vi "MultiFreqVelocityMove.vi"() -> ()   [LabVIEW 2022 SP3]
uses:
  <vilib>/Motion/FlexMotion/FunctionsVIs/Trajectory.llb/Load Acceleration/Deceleration.flx
  <vilib>/measure/NI_MAPro.lvlib
  <vilib>/Motion/FlexMotion/FunctionsVIs/StartStopMotion.llb/Start Motion (8 axes).flx
  <vilib>/Motion/FlexMotion/FunctionsVIs/StartStopMotion.llb/Stop Motion (8 axes).flx
  <vilib>/Utility/file.llb/Write Delimited Spreadsheet (DBL).vi
  <vilib>/Motion/FlexMotion/CustomControls/CustomControls.llb/Mask (8 axes).flx
  <vilib>/Motion/FlexMotion/FunctionsVIs/MotionIO.llb/Set Breakpoint Output MOMO (8 axes).flx
  <vilib>/Motion/FlexMotion/FunctionsVIs/Trajectory.llb/Wait for Move Complete (8 axes).flx
  <vilib>/Motion/FlexMotion/CustomControls/CustomControls.llb/AxisOrVectorSpace To Control.flx
panel:
  out "Final Position":i32
  out "Position":i32
  out "error out":errorcluster
  in  "Position Trigger Out?":bool=TRUE
  in  "Trigger every X Revolutions?":dbl=1.0
  in  "Filename":path=path "F:/test.txt"
  out "Filename Out":path=path "F:/test.txt"
  in  "Save Motor Velocities?":bool caption="Enable"
  in  "System Initilized?":bool
  in  "Stop":bool
  out "XY Graph":cluster{dbl[], dbl[]}[](graph)
  in  "Number of Components":i8=1 min=1 step=1
  in  "Seconds of Run Time":dbl=30.0
  in  "Counts Per (mm or rotation)":dbl=4000.0
  in  "Axis or Vector Space":T1=2 caption="Axis" items=["Axis 1"=1, "Axis 2"=2, "Axis 3"=3, "Axis 4"=4, "Axis 5"=5, "Axis 6"=6, "Axis 7"=7, "Axis 8"=8, "Vector Space 1"=17, "Vector Space 2"=18, "Vector Space 3"=19, "Vector Space 4"=20]
  in  "Component Phases":dbl[](array[numeric])=[0.0, 0.0, 0.0, 0.0] format="%.2p"
  in  "Component Speeds ((mm or rotations)/s)":dbl[](array[numeric])=[1.0, 0.25, 0.25, 1.0] format="%.2p"
  in  "Component Freqs (Hz)":dbl[](array[numeric])=[0.0, 5.0, 10.0, 400.0]
  in  "Run":bool
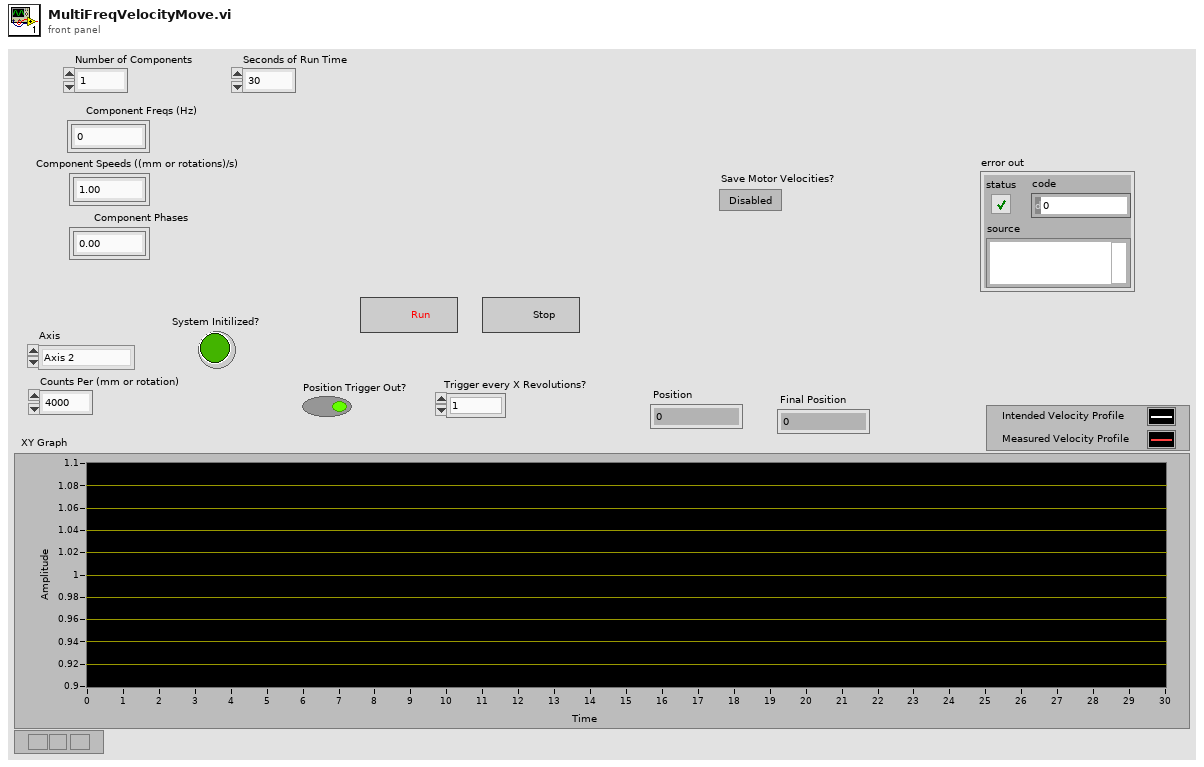
[diagram p1: front panel]
types:
  T1 = typedef "AxisOrVectorSpace To Control.flx" = u16
  T2 = typedef "Bd Id Out" = u8
  T3 = typedef "Mask (8 axes).flx" = cluster{"1":bool, "2":bool, "3":bool, "4":bool, "5":bool, "6":bool, "7":bool, "8":bool}
  T4 = enum16{"Absolute Position", "Relative Position", "Velocity", "Relative to Cap Pos", "Modulus Position", "Absolute Contouring", "Relative Contouring"}
  T5 = typedef "BoardID.ctl" = i32
  T6 = typedef "Resource Out (Enum).flx" = u16
  T7 = enum16{"No Change", "Reset on Breakpoint", "Set on Breakpoint", "Toggle on Breakpoint", "Create Pulse on Breakpoint"}
  T8 = enum16{"Absolute Breakpoint", "Relative Breakpoint", "Modulo Breakpoint", "Periodic Breakpoint"}
  T9 = enum16{"open", "replace", "create", "open or create", "replace or create", "replace or create with confirmation"}
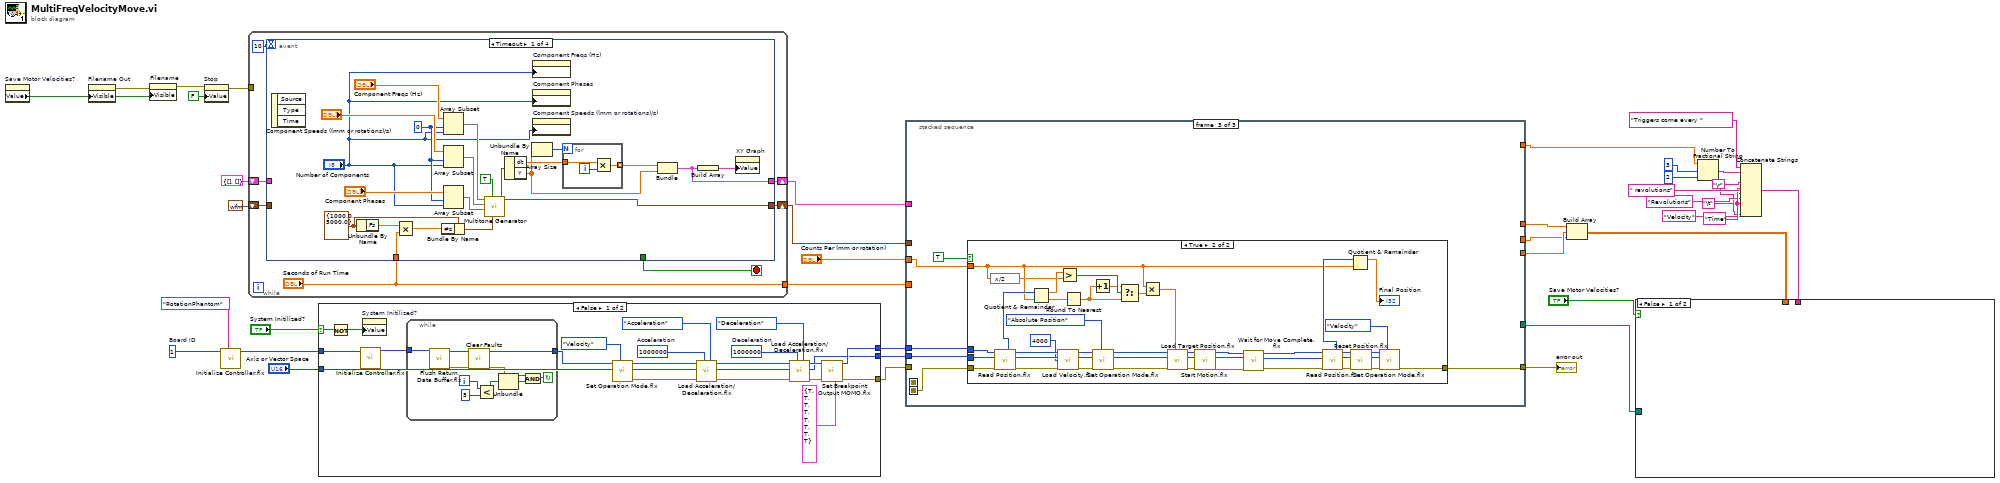
[diagram p0: block diagram]
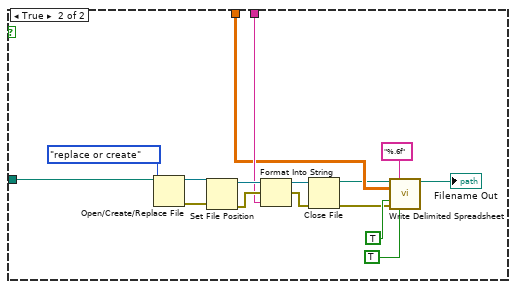
[diagram p2: hidden frame]
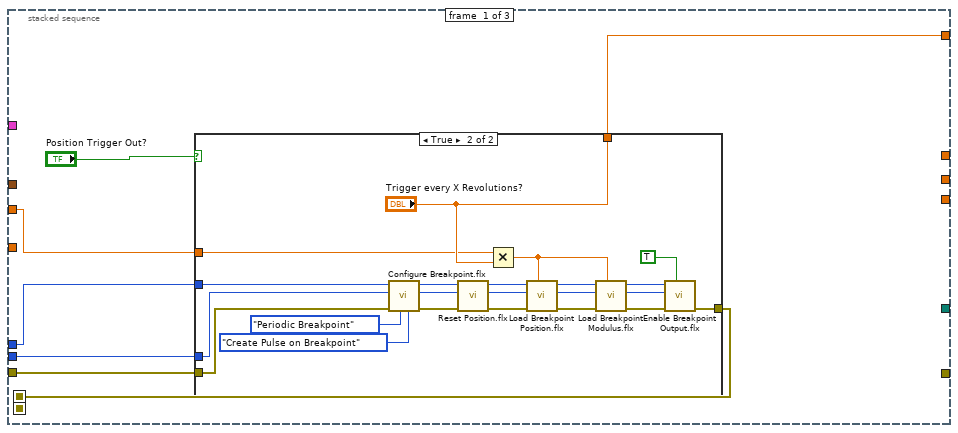
[diagram p3: hidden frame]
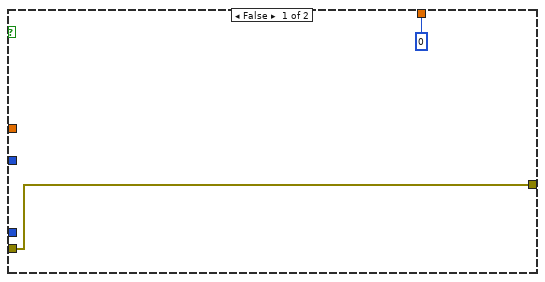
[diagram p4: hidden frame]
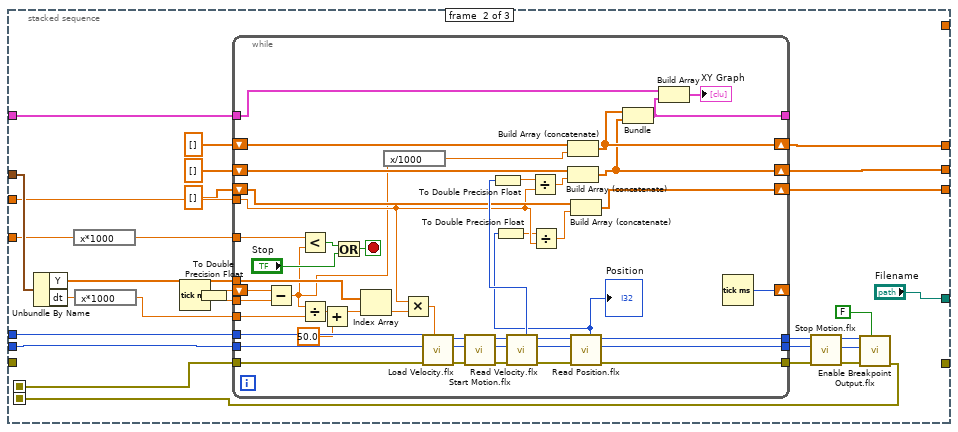
[diagram p5: hidden frame]
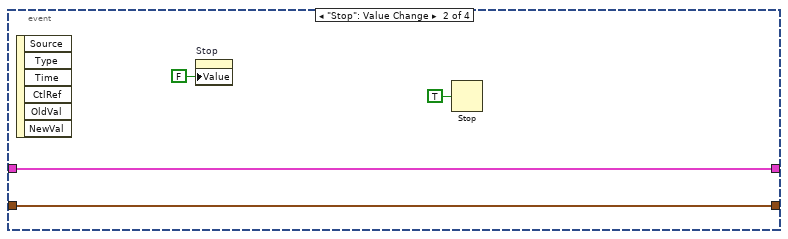
[diagram p8: hidden frame]
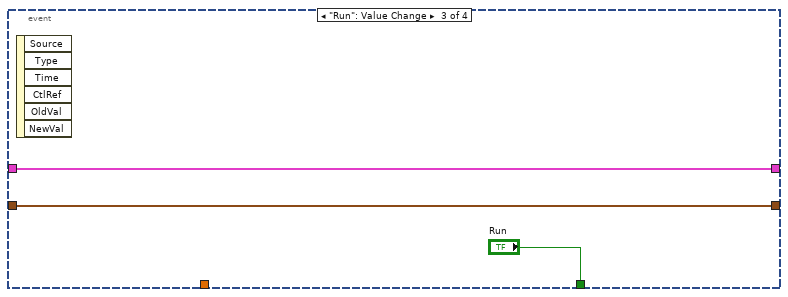
[diagram p9: hidden frame]
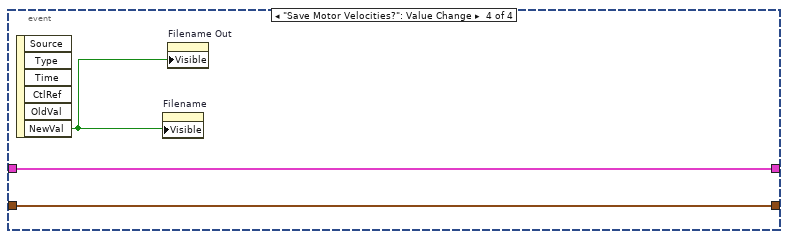
[diagram p10: hidden frame]
diagram:
  w8 = "\t"
  w9 = "\r"
  w2 = u8 1  # Board ID
  n1 = property on="Save Motor Velocities?" class="Bool (strict)"() -> ("Value"=w26:bool)  [unwired: 2 in, 2 out]
  n2 = property on="Filename Out" class="Path"("Visible"=w26) -> (error out=w25:errorcluster)  [unwired: 2 in, 1 out]
  n3 = property on="Filename" class="Path"(error in=w25, "Visible"=w26) -> (error out=w24:errorcluster)  [unwired: 1 in, 1 out]
  n4 = property on="Stop" class="Bool (strict)"(error in=w24, "Value"=FALSE ("Stop")) -> (error out=w14:errorcluster)  [unwired: 1 in, 1 out]
  n5 = call <vilib>:"Initialize Controller.flx"("Settings Name"="RotationPhantom", "Board ID"=w2) -> ("Bd ID Out"=w1:T2)  [unwired: 6 in, 1 out]
  n6 = while {
    tunnel: ["Seconds of Run Time"] -> w38
    shift-right: [w44] -> w36
    shift-left: cluster{dbl[], "Y":dbl[]} {[], "Y"=[]} -> [w43]
    shift-right: [w45] -> w37
    shift-left: waveform(dbl) {"t0"=timestamp(0 s since 1904-01-01), "dt"=1.0, "Y"=[]} ("signal out") -> [w42]
    tunnel: w14 -> [_]
    stop <- w40 stop-if-true
    n7 = event shown="[0] Timeout" {
      selector: _ -> [_ _ _ _]
      dyn-events: _ -> [_ _ _ _]
      timeout: 10 -> [_ _ _ _]
      tunnel: "Seconds of Run Time" -> [w46 _ _ _]
      tunnel: [w55 w73 w76 w79] -> w45
      tunnel: [w49 w72 w75 w78] -> w44
      tunnel: w43 -> [_ w72 w75 w78]
      tunnel: w42 -> [_ w73 w76 w79]
      tunnel: [_ _ "Run" _] -> w40
      event Timeout {
        w56 = 0 ("index")
        w63 = cluster{"Fs":dbl, "#s":dbl} {"Fs"=1000.0, "#s"=5000.0} ("sampling info")
        n8 = event-data() -> ()  [unwired: 1 in, 3 out]
        n9 = Unbundle By Name(w63) -> ("Fs"=w60:dbl)
        n10 = Multiply(x=w60, y=w46) -> (x*y=w62:dbl)
        n11 = Bundle By Name(cluster=w63, "#s"=w62) -> (w61:cluster{"Fs":dbl, "#s":dbl})
        n12 = Array Subset(array="Component Freqs (Hz)", index=w56, length="Number of Components") -> (w59:dbl[])
        n13 = Array Subset(array="Component Speeds ((mm or rotations)/s)", index=w56, length="Number of Components") -> (w58:dbl[])
        n14 = Array Subset(array="Component Phases", index=w56, length="Number of Components") -> (w57:dbl[])
        n15 = call <vilib>:"Multitone Generator.vi"("sampling info"=w61, "reset signal"=TRUE, "tone phases"=w57, "tone amplitudes"=w58, "tone frequencies"=w59) -> ("signal out"=w55:waveform(dbl))  [unwired: 3 in, 3 out]
        n16 = Unbundle By Name(w55) -> ("dt"=w54:dbl, "Y"=w50:dbl[])
        n17 = Array Size(array=w50) -> (size(s)=w51:i32)
        n18 = property on="Component Freqs (Hz)" class="Arr (strict)"("Number of Columns"="Number of Components") -> ()  [unwired: 2 in, 2 out]
        n19 = property on="Component Phases" class="Arr (strict)"("Number of Columns"="Number of Components") -> ()  [unwired: 2 in, 2 out]
        n20 = property on="Component Speeds ((mm or rotations)/s)" class="Arr (strict)"("Number of Columns"="Number of Components") -> ()  [unwired: 2 in, 2 out]
        n21 = for {
          N: w51 -> [_]
          tunnel: w54 -> [w68]
          tunnel: [w67] -> w53 mode=indexing
          i -> [w69]
          n22 = Multiply(x=w68, y=w69) -> (x*y=w67:dbl)
        }
        n23 = Bundle(w53, "Y"=w50) -> (w49:cluster{dbl[], "Y":dbl[]})  [unwired: 1 in]
        n24 = Build Array(w49) -> (w52:cluster{dbl[], "Y":dbl[]}[])
        n25 = property on="XY Graph" class="XYGraph (strict)"("Value"=w52) -> ()  [unwired: 2 in, 2 out]
      }
      event "Stop": Value Change {
        n26 = event-data() -> ()  [unwired: 1 in, 6 out]
        n27 = property on="Stop" class="Bool (strict)"("Value"=FALSE ("Stop")) -> ()  [unwired: 2 in, 2 out]
        n28 = Stop(stop? (T)=TRUE) -> ()
      }
      event "Run": Value Change {
        n29 = event-data() -> ()  [unwired: 1 in, 6 out]
      }
      event "Save Motor Velocities?": Value Change {
        n30 = event-data() -> ("NewVal"=w77:bool)  [unwired: 1 in, 5 out]
        n31 = property on="Filename" class="Path"("Visible"=w77) -> ()  [unwired: 2 in, 2 out]
        n32 = property on="Filename Out" class="Path"("Visible"=w77) -> ()  [unwired: 2 in, 2 out]
      }
    }
  }
  n33 = case shown="False" "System Initilized?" {
    selector: "System Initilized?" -> [w102 _]
    tunnel: [w83 w114] -> w31
    tunnel: "Axis or Vector Space" -> [w86 w114]
    tunnel: w1 -> [w100 w113]
    tunnel: [w84 w113] -> w32
    tunnel: [w80 _] -> w30
    frame False {
      w94 = u32 1000000  # Deceleration
      w93 = u32 1000000  # Acceleration
      n34 = Not(x=w102) -> (.not. x?=w101:bool)
      n35 = call <vilib>:"Initialize Controller.flx"("Board ID"=w100) -> ("Bd ID Out"=w99:T2)  [unwired: 7 in, 1 out]
      n36 = property on="System Initilized?" class="Bool (strict)"("Value"=w101) -> ()  [unwired: 2 in, 2 out]
      n37 = while {
        tunnel: w99 -> [w112]
        tunnel: [w110] -> w87
        i -> [w105]
        stop <- w106 continue-if-true
        n38 = call <vilib>:"Flush Return Data Buffer.flx"("Board ID"=w112) -> ("error out"=w108:errorcluster, "Bd ID Out"=w111:T2)  [unwired: 6 in]
        n39 = call <vilib>:"Clear Faults.vi"("error in (no error)"=w108, "board in"=w111) -> ("error out"=w109:errorcluster, "board out"=w110:T5)  [unwired: 8 in]
        n40 = Less?(x=w105, y=5) -> (x < y?=w104:bool)
        n41 = Unbundle(w109) -> ("status"=w107:bool)  [unwired: 2 out]
        n42 = And(x=w107, y=w104) -> (x .and. y?=w106:bool)
      }
      n43 = call <vilib>:"Set Operation Mode.flx"("Position Mode (Absolute)"=T4."Velocity", "Axis or Vector Space"=w86, "Board ID"=w87) -> ("error out"=w98:errorcluster, "Resource Output"=w96:T6, "Bd ID Out"=w97:T2)  [unwired: 3 in]
      n44 = call "Load Acceleration/Deceleration.flx"("Acceleration Type (Both)"=enum16{"Both", "Acceleration", "Deceleration"}."Acceleration", "Acceleration (100000)"=w93, "error in (no error)"=w98, "Axis or Vector Space"=w96, "Board ID"=w97) -> ("error out"=w90:errorcluster, "Resource Output"=w88:T6, "Bd ID Out"=w89:T2)  [unwired: 2 in]
      n45 = call "Load Acceleration/Deceleration.flx"("Acceleration Type (Both)"=enum16{"Both", "Acceleration", "Deceleration"}."Deceleration", "Acceleration (100000)"=w94, "error in (no error)"=w90, "Axis or Vector Space"=w88, "Board ID"=w89) -> ("error out"=w81:errorcluster, "Resource Output"=w83:T6, "Bd ID Out"=w85:T2)  [unwired: 2 in]
      n46 = call-poly <vilib>:"Set Breakpoint Output MOMO.flx"("Must Off (False)"=T3 {"1"=TRUE, "2"=TRUE, "3"=TRUE, "4"=TRUE, "5"=TRUE, "6"=TRUE, "7"=TRUE, "8"=TRUE}, "error in (no error)"=w81, "Board ID"=w85) -> ("error out"=w80:errorcluster, "Bd ID Out"=w84:T2)  [unwired: 3 in, 2 out]
    }
    frame True {
    }
  }
  n47 = stacked-sequence {
    seq-local: [w115 _ _] -> [_ w150 _]
    seq-local: [_ w146 _] -> [_ _ w223]
    tunnel: w37 -> [_ w173 _]
    tunnel: w32 -> [w121 w148 w226]
    tunnel: w31 -> [w120 w147 w225]
    tunnel: w30 -> [w119 _ _]
    tunnel: w38 -> [_ w169 _]
    tunnel: w36 -> [_ w165 _]
    tunnel: "Counts Per (mm or rotation)" -> [w116 w163 w224]
    tunnel: [_ w160 _] -> w23
    tunnel: [_ w159 _] -> w21
    tunnel: [_ w152 _] -> w22
    tunnel: [w117 _ _] -> w19
    tunnel: [_ "Filename" _] -> w6
    tunnel: [_ _ w222] -> w4
    frame #0 {
      n48 = case shown="True" "Position Trigger Out?" {
        tunnel: w121 -> [_ w125]
        tunnel: w120 -> [_ w124]
        tunnel: w119 -> [w122 w140]
        tunnel: [0 ("Breakpoint Modolus") "Trigger every X Revolutions?"] -> w117
        tunnel: w116 -> [_ w127]
        tunnel: [w122 w126] -> w115
        frame False {
        }
        frame True {
          n49 = call <vilib>:"Configure Breakpoint.flx"("Action (No Change)"=T7."Create Pulse on Breakpoint", "Mode (Absolute)"=T8."Periodic Breakpoint", "error in (no error)"=w140, "Axis or Encoder"=w124, "Board ID"=w125) -> ("error out"=w134:errorcluster, "Resource Output"=w135:T6, "Bd ID Out"=w138:T2)  [unwired: 4 in]
          n50 = call <vilib>:"Reset Position.flx"("error in (no error)"=w134, "Axis"=w135, "Board ID"=w138) -> ("error out"=w133:errorcluster, "Resource Output"=w136:T6, "Bd ID Out"=w137:T2)  [unwired: 4 in]
          n51 = Multiply(x=w127, y="Trigger every X Revolutions?") -> (x*y=w128:dbl)
          n52 = call <vilib>:"Load Breakpoint Position.flx"("Breakpoint Position (0)"=w128, "error in (no error)"=w133, "Axis or Encoder"=w136, "Board ID"=w137) -> ("error out"=w139:errorcluster, "Resource Output"=w143:T6, "Bd ID Out"=w144:T2)  [unwired: 3 in]
          n53 = call <vilib>:"Load Breakpoint Modulus.flx"("Breakpoint Modulus (0)"=w128, "error in (no error)"=w139, "Axis or Encoder"=w143, "Board ID"=w144) -> ("error out"=w145:errorcluster, "Resource Output"=w141:T6, "Bd ID Out"=w142:T2)  [unwired: 3 in]
          n54 = call <vilib>:"Enable Breakpoint Output.flx"("Enable Breakpoint"=TRUE, "error in (no error)"=w145, "Axis or Encoder"=w141, "Board ID"=w142) -> ("error out"=w126:errorcluster)  [unwired: 3 in, 2 out]
        }
      }
    }
    frame #1 {
      n55 = Unbundle By Name(w173) -> ("Y"=w166:dbl[], "dt"=w161:dbl)
      n56 = expression code="x*1000"(w169) -> (w168:dbl)
      n57 = expression code="x*1000"(w161) -> (w167:dbl)
      n58 = Tick Count (ms)() -> (millisecond timer value=w170:u32)
      n59 = To Double Precision Float(number=w170) -> (double precision float=w149:dbl)
      n60 = while {
        tunnel: [w185] -> w171
        tunnel: [w184] -> w172
        tunnel: w150 -> [w216]
        tunnel: w147 -> [w220]
        tunnel: w148 -> [w190]
        tunnel: w166 -> [w215]
        tunnel: w167 -> [w211]
        shift-right: [w214] -> _
        shift-left: w149 -> [w213]
        tunnel: w149 -> [w212]
        tunnel: w168 -> [w208]
        tunnel: w165 -> [w203]
        shift-right: [w198] -> w160
        shift-left: dbl[] [] -> [w202]
        shift-right: [w197] -> w159
        shift-left: dbl[] [] -> [w201]
        tunnel: w163 -> [w180]
        tunnel: [w191] -> _
        tunnel: [w186] -> w154
        shift-right: [w183] -> w152
        shift-left: dbl[] [] -> [w182]
        stop <- w194 stop-if-true
        n61 = Subtract(x=w213, y=w212) -> (x-y=w176:dbl)
        n62 = Less?(x=w208, y=w176) -> (x < y?=w209:bool)
        n63 = Divide(x=w176, y=w211) -> (x/y=w195:dbl)
        n64 = Add(x=w195, y=50.0) -> (x+y=w178:dbl)
        n65 = Or(x=w209, y="Stop") -> (x .or. y?=w194:bool)
        n66 = Index Array(array=w215, index=w178) -> (element=w210:dbl)
        n67 = expression code="x/1000"(w176) -> (w192:dbl)
        n68 = Multiply(x=w180, y=w210) -> (x*y=w204:dbl)
        n69 = call <vilib>:"Load Velocity.flx"("Velocity (10000)"=w204, "error in (no error)"=w216, "Axis or Vector Space"=w220, "Board ID"=w190) -> ("error out"=w217:errorcluster, "Resource Output"=w219:T6, "Bd ID Out"=w218:T2)  [unwired: 3 in]
        n70 = call-poly <vilib>:"Start Motion.flx"("error in (no error)"=w217, "Axis or Vector Space"=w219, "Board ID"=w218) -> ("error out"=w205:errorcluster, "Resource Output"=w206:T6, "Bd ID Out"=w207:T2)  [unwired: 3 in]
        n71 = call <vilib>:"Read Velocity.flx"("error in (no error)"=w205, "Axis or Vector Space"=w206, "Board ID"=w207) -> ("error out"=w187:errorcluster, "Resource Output"=w188:T6, "Bd ID Out"=w189:T2, "Filtered Velocity"=w196:i32)  [unwired: 3 in]
        n72 = To Double Precision Float(number=w196) -> (double precision float=w175:dbl)
        n73 = Divide(x=w175, y=w180) -> (x/y=w200:dbl)
        n74 = Build Array (concatenate)(w202, w192) -> (w198:dbl[])
        n75 = Build Array (concatenate)(w201, w200) -> (w197:dbl[])
        n76 = call <vilib>:"Read Position.flx"("error in (no error)"=w187, "Axis"=w188, "Board ID"=w189) -> ("error out"=w186:errorcluster, "Resource Output"=w185:T6, "Bd ID Out"=w184:T2, "Position"=w179:i32)  [unwired: 3 in]
        "Position" <- w179
        n77 = To Double Precision Float(number=w179) -> (double precision float=w174:dbl)
        n78 = Divide(x=w174, y=w180) -> (x/y=w181:dbl)
        n79 = Build Array (concatenate)(w182, w181) -> (w183:dbl[])
        n80 = Bundle(w198, w197) -> (w191:cluster{dbl[], dbl[]})  [unwired: 1 in]
        n81 = Build Array(w203, w191) -> (→"XY Graph":cluster{dbl[], "Y":dbl[]}[])
        n82 = Tick Count (ms)() -> (millisecond timer value=w214:u32)
      }
      n83 = call-poly <vilib>:"Stop Motion.flx"("error in (no error)"=w154, "Axis or Vector Space"=w171, "Board ID"=w172) -> ("error out"=w156:errorcluster, "Resource Output"=w157:T6, "Bd ID Out"=w158:T2)  [unwired: 4 in]
      n84 = call <vilib>:"Enable Breakpoint Output.flx"("Enable Breakpoint"=FALSE, "error in (no error)"=w156, "Axis or Encoder"=w157, "Board ID"=w158) -> ("error out"=w146:errorcluster)  [unwired: 3 in, 2 out]
    }
    frame #2 {
      n85 = case shown="True" TRUE {
        tunnel: w226 -> [_ w269]
        tunnel: w225 -> [_ w268]
        tunnel: w224 -> [_ w238]
        tunnel: w223 -> [w227 w242]
        tunnel: [w227 w241] -> w222
        frame False {
        }
        frame True {
          n86 = expression code="x/2"(w238) -> (w237:dbl)
          n87 = call <vilib>:"Read Position.flx"("error in (no error)"=w242, "Axis"=w268, "Board ID"=w269) -> ("error out"=w255:errorcluster, "Resource Output"=w251:T6, "Bd ID Out"=w256:T2, "Position"=w267:i32)  [unwired: 3 in]
          n88 = Quotient & Remainder(x=w267, y=w238) -> (x-y*floor(x/y)=w239:dbl, floor(x/y)=w240:dbl)
          n89 = call <vilib>:"Load Velocity.flx"("Velocity (10000)"=4000, "error in (no error)"=w255, "Axis or Vector Space"=w251, "Board ID"=w256) -> ("error out"=w253:errorcluster, "Resource Output"=w252:T6, "Bd ID Out"=w254:T2)  [unwired: 3 in]
          n90 = Greater?(x=w239, y=w237) -> (0:w235:bool)
          n91 = Round To Nearest(number=w240) -> (nearest integer value=w234:dbl)
          n92 = Increment(x=w234) -> (x+1=w233:dbl)
          n93 = call <vilib>:"Set Operation Mode.flx"("Position Mode (Absolute)"=T4."Absolute Position", "error in (no error)"=w253, "Axis or Vector Space"=w252, "Board ID"=w254) -> ("error out"=w259:errorcluster, "Resource Output"=w263:T6, "Bd ID Out"=w266:T2)  [unwired: 2 in]
          n94 = Select(t=w233, s=w235, f=w234) -> (s? t:f=w236:dbl)
          n95 = Multiply(x=w238, y=w236) -> (x*y=w248:dbl)
          n96 = call <vilib>:"Load Target Position.flx"("Target Position (0)"=w248, "error in (no error)"=w259, "Axis"=w263, "Board ID"=w266) -> ("error out"=w258:errorcluster, "Resource Output"=w264:T6, "Bd ID Out"=w265:T2)  [unwired: 3 in]
          n97 = call-poly <vilib>:"Start Motion.flx"("error in (no error)"=w258, "Axis or Vector Space"=w264, "Board ID"=w265) -> ("error out"=w228:errorcluster, "Resource Output"=w231:T6, "Bd ID Out"=w257:T2)  [unwired: 3 in]
          n98 = call-poly <vilib>:"Wait for Move Complete.flx"("error in (no error)"=w228, "Axis or Vector Space"=w231, "Board ID"=w257) -> ("error out"=w229:errorcluster, "Resource Output"=w230:T6, "Bd ID Out"=w232:T2)  [unwired: 5 in, 1 out]
          n99 = call <vilib>:"Read Position.flx"("error in (no error)"=w229, "Axis"=w230, "Board ID"=w232) -> ("error out"=w243:errorcluster, "Resource Output"=w244:T6, "Bd ID Out"=w245:T2, "Position"=w247:i32)  [unwired: 3 in]
          n100 = Quotient & Remainder(x=w247, y=w238) -> (x-y*floor(x/y)=→"Final Position":dbl)  [unwired: 1 out]
          n101 = call <vilib>:"Reset Position.flx"("error in (no error)"=w243, "Axis"=w244, "Board ID"=w245) -> ("error out"=w260:errorcluster, "Resource Output"=w249:T6, "Bd ID Out"=w261:T2)  [unwired: 4 in]
          n102 = call <vilib>:"Set Operation Mode.flx"("Position Mode (Absolute)"=T4."Velocity", "error in (no error)"=w260, "Axis or Vector Space"=w249, "Board ID"=w261) -> ("error out"=w241:errorcluster)  [unwired: 2 in, 2 out]
        }
      }
    }
  }
  "error out" <- w4
  n103 = Build Array(w23, w22, w21) -> (w7:dbl[][])
  n104 = Number To Fractional String(number=w19, width (-)=i16 3, precision (6)=i16 2) -> (F-format string=w17:string)  [unwired: 1 in]
  n105 = Concatenate Strings("Triggers come every " ("Comment"), w17, " revolutions" ("string"), w9, "Time" ("string"), w8, "Revolutions" ("string"), w8, "Velocity" ("string"), w9) -> (w13:string)
  n106 = case shown="False" "Save Motor Velocities?" {
    tunnel: w13 -> [_ w282]
    tunnel: w7 -> [_ w278]
    tunnel: w6 -> [_ w271]
    frame False {
    }
    frame True {
      n107 = Open/Create/Replace File(file path (use dialog)=w271, operation (0:open)=T9."replace or create") -> (refnum out=w285:refnum<file>, error out=w286:errorcluster)  [unwired: 4 in, 1 out]
      n108 = Set File Position(refnum=w285, error in=w286) -> (refnum out=w283:refnum<file>, error out=w284:errorcluster)  [unwired: 2 in]
      n109 = Format Into String(initial string=w283, error in=w284, w282) -> (resulting string=w280:refnum<file>, error out=w281:errorcluster)  [unwired: 1 in]
      n110 = Close File(refnum=w280, error in=w281) -> (path=w275:path, error out=w274:errorcluster)
      n111 = call-poly <vilib>:"Write Delimited Spreadsheet.vi"("file path (dialog if empty)"=w275, "format (%.3f)"="%.6f", "2D data"=w278, "append to file? (new file:F)"=TRUE, "error in (no error)"=w274, "transpose? (no:F)"=TRUE) -> ("new file path (Not A Path if cancelled)"=→"Filename Out":path)  [unwired: 8 in, 1 out]
    }
  }
